vi "Set_not_connect.vi"(10 "Z_HSwitch_state 2":T1={"Write"=FALSE, "Z1_ind visu"=5, "Z1_ind_blinking"=FALSE, "Z_HSwitch_out"=FALSE, "Z_HSwitch_visible"=FALSE, "Z_HSwitch_disabled"=enum."Enabled"}) -> (1 "reset_timer":bool, 2 "Z_HSwitch_state":T1, 3 "Z1_ind_state":T2, 4 "load_timer":bool)   [LabVIEW 2019]
uses:
  Button state.ctl
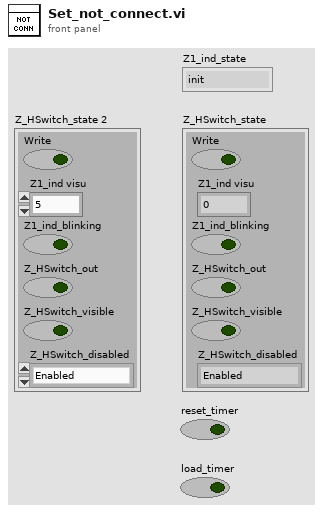
[diagram p1: front panel]
types:
  T1 = cluster{"Write":bool, "Z1_ind visu":u8, "Z1_ind_blinking":bool, "Z_HSwitch_out":bool, "Z_HSwitch_visible":bool, "Z_HSwitch_disabled":enum8{"Enabled", "Disabled", "Disabled and Grayed Out"}}
  T2 = typedef "Button state.ctl" = enum16{"init", "not connect", "local disabled", "local hand", "set hand", "hand", "set auto", "auto", "dist"}
  T3 = enum8{"Enabled", "Disabled", "Disabled and Grayed Out"}
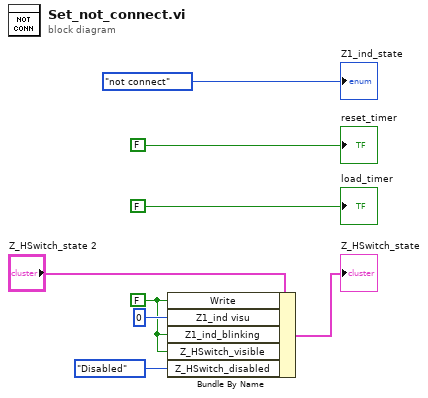
[diagram p0: block diagram]
diagram:
  w6 = FALSE ("Z_ASwitch")
  n1 = Bundle By Name(cluster="Z_HSwitch_state 2", "Write"=w6, "Z1_ind visu"=u8 0, "Z1_ind_blinking"=w6, "Z_HSwitch_visible"=w6, "Z_HSwitch_disabled"=T3."Disabled" ("Disabled")) -> (→"Z_HSwitch_state":T1)
  "Z1_ind_state" <- Button_state."not connect" ("Z1_State")
  "load_timer" <- FALSE ("Z_ASwitch")
  "reset_timer" <- FALSE ("Z_ASwitch")
